vi "USB6343_initialize.vi"() -> (0 "error out":errorcluster caption="错误输出", 3 "tasks":T1)   [LabVIEW 2013]
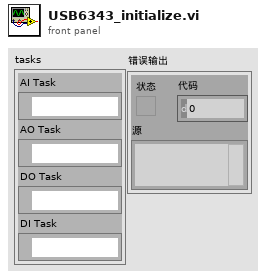
[diagram p1: front panel]
types:
  T1 = cluster{"AI Task":refnum<k21>, "AO Task":refnum<k21>, "DO Task":refnum<k21>, "DI Task":refnum<k21>}
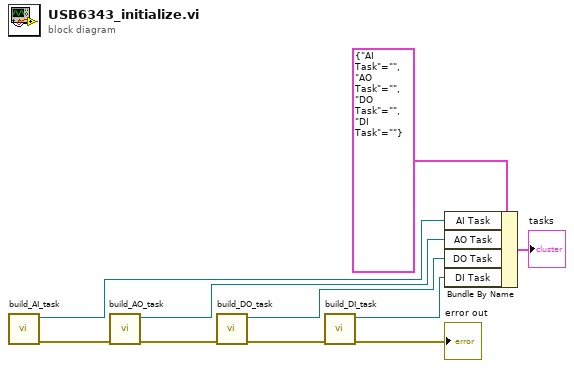
[diagram p0: block diagram]
diagram:
  n1 = call "build_AI_task.vi"() -> ("error out"=w7:errorcluster, "task out"=w9:refnum<k21>)  [unwired: 10 in]
  n2 = call "build_AO_task.vi"("error in"=w7) -> ("error out"=w3:errorcluster, "task out"=w8:refnum<k21>)  [unwired: 9 in]
  n3 = call "build_DO_task.vi"("error in"=w3) -> ("error out"=w2:errorcluster, "task out"=w1:refnum<k21>)  [unwired: 9 in]
  n4 = call "build_DI_task.vi"("error in"=w2) -> ("error out"=→"error out":errorcluster, "task out"=w6:refnum<k21>)  [unwired: 9 in]
  n5 = Bundle By Name(cluster=T1 {"AI Task"="", "AO Task"="", "DO Task"="", "DI Task"=""}, "AI Task"=w9, "AO Task"=w8, "DO Task"=w1, "DI Task"=w6) -> (→"tasks":T1)
